vi "string to reading.vi"(8 "error in (no error)":errorcluster, 11 "binary string":string) -> (0 "error out":errorcluster, 3 "reading":T1)   [LabVIEW 2017]
uses:
  typedefs/reading.ctl
  typedefs/readingType.ctl
panel:
  out "length 4":i32
  out "length 3":i32
  out "length 2":i32
  out "length":i32
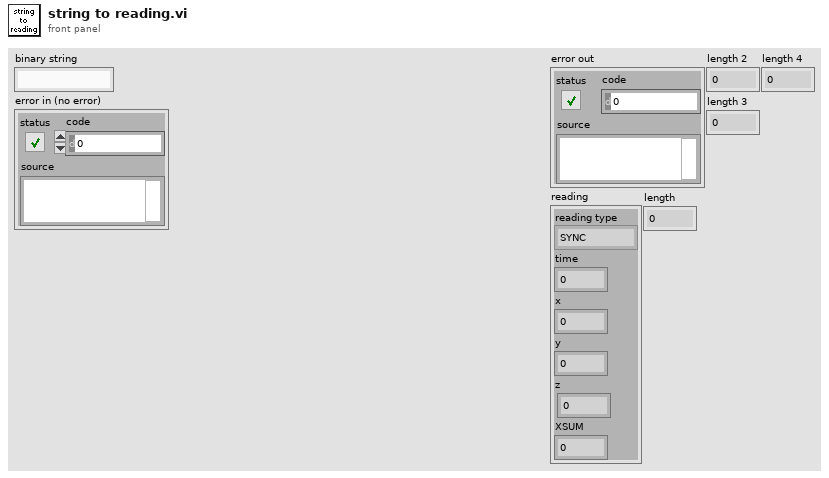
[diagram p1: front panel]
types:
  T1 = typedef "reading.ctl" = cluster{"reading type":T2, "time":fxp<+,48,48>, "x":sgl, "y":sgl, "z":sgl, "XSUM":u8}
  T2 = typedef "readingType.ctl" = enum8{"SYNC", "DETVAL", "COILI", "MAGVEC", "ACCVEC"}
  T3 = enum16{"big-endian, network order", "native, host order", "little-endian"}
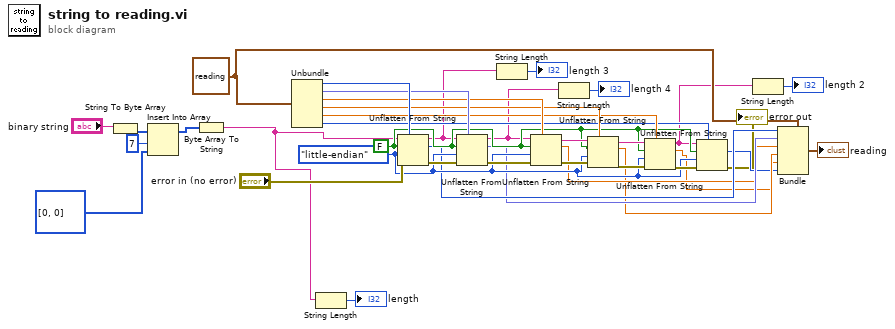
[diagram p0: block diagram]
diagram:
  w23 = T3."little-endian" ("byte order (0:big-endian, network order)")
  w24 = FALSE ("data includes array or string size? (T)")
  w22 = T1 {"reading type"=enum."SYNC", "time"=0.0, "x"=0.0, "y"=0.0, "z"=0.0, "XSUM"=0} ("reading")
  n1 = String To Byte Array(string="binary string") -> (unsigned byte array=w5:u8[])
  n2 = Insert Into Array(array=w5, index=7, new element=u8[] [0, 0]) -> (w2:u8[])
  n3 = Byte Array To String(unsigned byte array=w2) -> (string=w1:string)
  n4 = Unbundle(w22) -> ("reading type"=w38:T2, "time"=w37:fxp<+,48,48>, "x"=w33:sgl, "y"=w32:sgl, "z"=w29:sgl, "XSUM"=w26:u8)
  n5 = String Length(string=w1) -> (length=→"length":i32)
  n6 = Unflatten From String(type=w38, binary string=w1, data includes array or string size? (T)=w24, byte order (0:big-endian, network order)=w23, error in (no error)="error in (no error)") -> (rest of the binary string=w10:string, value=w21:T2, error out=w36:errorcluster)
  n7 = Unflatten From String(type=w37, binary string=w10, data includes array or string size? (T)=w24, byte order (0:big-endian, network order)=w23, error in (no error)=w36) -> (rest of the binary string=w8:string, value=w20:fxp<+,48,48>, error out=w34:errorcluster)
  n8 = String Length(string=w10) -> (length=→"length 3":i32)
  n9 = Unflatten From String(type=w33, binary string=w8, data includes array or string size? (T)=w24, byte order (0:big-endian, network order)=w23, error in (no error)=w34) -> (rest of the binary string=w31:string, value=w19:sgl, error out=w30:errorcluster)
  n10 = String Length(string=w8) -> (length=→"length 4":i32)
  n11 = Unflatten From String(type=w32, binary string=w31, data includes array or string size? (T)=w24, byte order (0:big-endian, network order)=w23, error in (no error)=w30) -> (rest of the binary string=w28:string, value=w18:sgl, error out=w27:errorcluster)
  n12 = Unflatten From String(type=w29, binary string=w28, data includes array or string size? (T)=w24, byte order (0:big-endian, network order)=w23, error in (no error)=w27) -> (rest of the binary string=w12:string, value=w17:sgl, error out=w25:errorcluster)
  n13 = Unflatten From String(type=w26, binary string=w12, data includes array or string size? (T)=w24, byte order (0:big-endian, network order)=w23, error in (no error)=w25) -> (value=w16:u8, error out=→"error out":errorcluster)  [unwired: 1 out]
  n14 = String Length(string=w12) -> (length=→"length 2":i32)
  n15 = Bundle(cluster=w22, "reading type"=w21, "time"=w20, "x"=w19, "y"=w18, "z"=w17, "XSUM"=w16) -> (→"reading":T1)
